vi "Instr_InitObject.vi"(8 "error in (no error)":errorcluster, 9 "Instrument Configuration":variant, 10 "Instrument address":refnum<visa-resource-name>, 11 "Pickering in":refnum<class "Pickering.lvclass">) -> (0 "error out":errorcluster, 3 "Pickering out":refnum<class "Pickering.lvclass">)   [LabVIEW 2018, in "Pickering.lvclass"]
uses:
  Pickering.lvclass
  InstrumentSetup.vi
  PickeringMUX_CommandsGlobal.vi
  PickeringMatrix_CommandsGlobal.vi
  Switching.lvclass
  InstrControl.lvclass
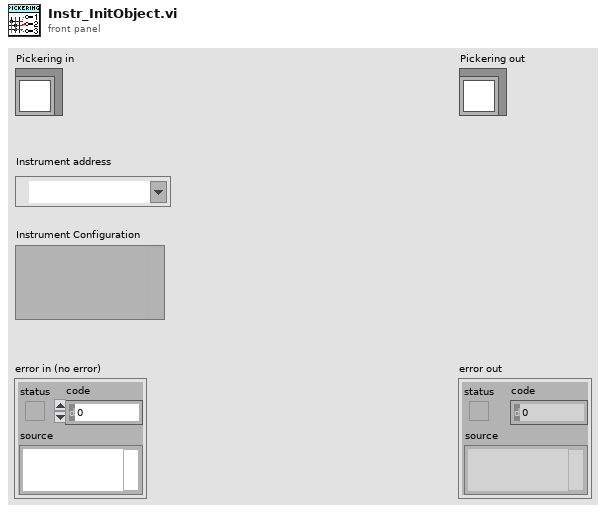
[diagram p1: front panel]
types:
  T1 = cluster{"Matrix address":string, "Mux1 address":string, "Mux2 address":string, "Pickering":refnum<class "Pickering.lvclass">, "Matrix X Channels":cluster{"Bias Supply / SMU LO":i32, "Bias Supply / SMU HI":i32, "CV Box LO":i32, "CV Box HI":i32, "CV Box LO IN":i32, "CV Box HI IN":i32, "Volt meter LO":i32, "Volt meter HI":i32, "Mux1 C1":i32, "Mux1 C2":i32, "Mux2 C1":i32, "Mux2 C2":i32}}
  T2 = cluster{"Matrix address":string, "Instrument name":string, "Instrument type":u16, "Command \"Matrix Reset\"":string, "Command \"Connect Matrix Channels\"":string, "Command \"Disconnect Matrix Channels\"":string}
  T3 = cluster{"Mux1 address":string, "Mux2 address":string, "Instrument name":string, "Instrument type":u16, "Command \"MUX Reset\"":string, "Command \"Select MUX Channel\"":string}
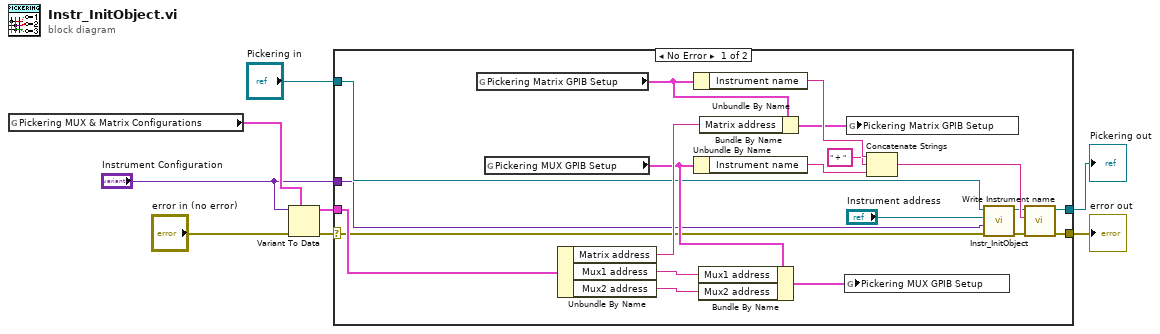
[diagram p0: block diagram]
diagram:
  n1 = global read "InstrumentSetup.vi" "Pickering MUX & Matrix Configurations"() -> (w3:T1)
  n2 = Variant To Data(error in="error in (no error)", type=w3, Variant="Instrument Configuration") -> (data=w2:T1, error out=w4:errorcluster)
  n3 = case shown="No Error" w4 {
    selector: w4 -> [w15 w30]
    tunnel: [w9 w30] -> w6
    tunnel: "Pickering in" -> [w16 w29]
    tunnel: [w10 w29] -> w7
    tunnel: w2 -> [w17 _]
    tunnel: "Instrument Configuration" -> [w11 _]
    frame No Error {
      n4 = global read "PickeringMatrix_CommandsGlobal.vi" "Pickering Matrix GPIB Setup"() -> (w20:T2)
      n5 = global read "PickeringMUX_CommandsGlobal.vi" "Pickering MUX GPIB Setup"() -> (w21:T3)
      n6 = Unbundle By Name(w17) -> ("Matrix address"=w24:string, "Mux1 address"=w23:string, "Mux2 address"=w22:string)
      n7 = Unbundle By Name(w20) -> ("Instrument name"=w28:string)
      n8 = Unbundle By Name(w21) -> ("Instrument name"=w27:string)
      n9 = Bundle By Name(cluster=w21, "Mux1 address"=w23, "Mux2 address"=w22) -> (w19:T3)
      n10 = Bundle By Name(cluster=w20, "Matrix address"=w24) -> (w18:T2)
      n11 = global write "PickeringMUX_CommandsGlobal.vi" "Pickering MUX GPIB Setup"(w19) -> ()
      n12 = global write "PickeringMatrix_CommandsGlobal.vi" "Pickering Matrix GPIB Setup"(w18) -> ()
      n13 = Concatenate Strings(w28, " + ", w27) -> (w25:string)
      n14 = call-parent "Instr_InitObject.vi"("error in (no error)"=w15, "Instrument Configuration"=w11, "Instrument address"="Instrument address", "Switching in"=w16) -> ("error out"=w14:errorcluster, "Switching out"=w13:refnum<class "Pickering.lvclass">)  [unwired: 6 in]
      n15 = call-dynamic "Write Instrument name.vi"("error in (no error)"=w14, "Instrument name"=w25, "InstControl in"=w13) -> ("error out"=w9:errorcluster, "InstControl out"=w10:refnum<class "Pickering.lvclass">)  [unwired: 7 in]
    }
    frame Error {
    }
  }
  "error out" <- w6
  "Pickering out" <- w7
